vi "get_transport_error.vi"(8 "error in (no error)":errorcluster, 11 "Request in":refnum<class "Request.lvclass">) -> (0 "error out":errorcluster, 2 "transport_error":string, 3 "Request in":refnum<class "Request.lvclass">)   [LabVIEW 2020, in "reqwest.lvlib" / "Request.lvclass"]
uses:
  Request.lvclass
  Request.lvclass/Request.ctl
  reqwest.lvlib
  lv_reqwest_32.dll
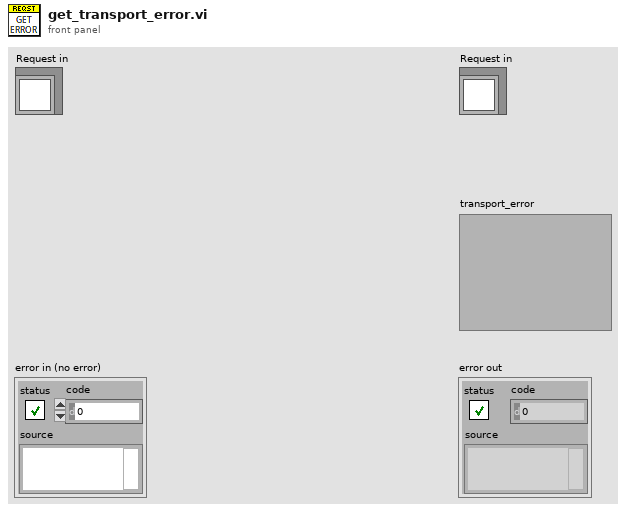
[diagram p1: front panel]
types:
  T1 = typedef "reqwest.lvlib/Request.lvclass/request_id.ctl" = u64
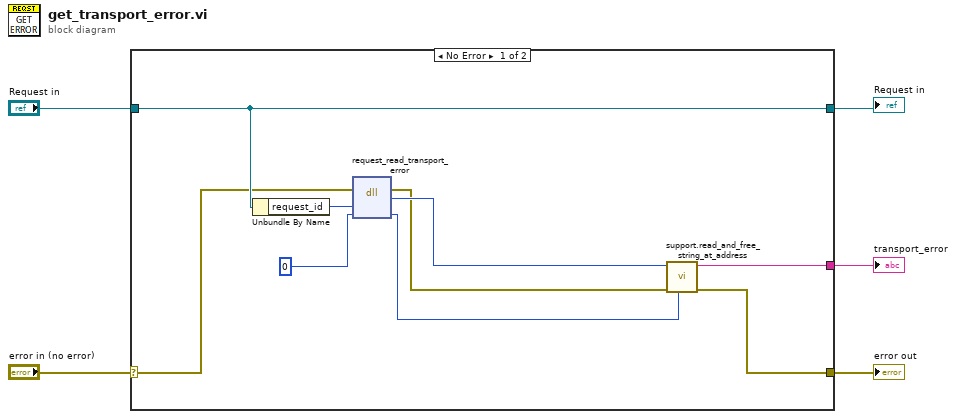
[diagram p0: block diagram]
diagram:
  n1 = case shown="No Error" "error in (no error)" {
    selector: "error in (no error)" -> [w9 w15]
    tunnel: "Request in" -> [w10 w16]
    tunnel: [w11 _] -> w3
    tunnel: [w8 w15] -> w1
    tunnel: [w10 w16] -> w2
    frame No Error {
      n2 = Unbundle By Name(w10) -> ("request_id"=w12:T1)
      n3 = dll-call lib="C:/Projects/reqwest-rs-labview/lv_src/lv_reqwest_*.*" fn="request_read_transport_error"(error in=w9, "request_id"=w12, "num_bytes"=u32 0) -> (error out=w13:errorcluster, "string_ptr"=w14:u64, "num_bytes"=w6:u32)  [unwired: 3 in, 1 out]
      n4 = call "support.read_and_free_string_at_address.vi"("string_length"=w6, "error in (no error)"=w13, "string_ptr"=w14) -> ("error out"=w8:errorcluster, "string"=w11:string)  [unwired: 7 in]
    }
    frame Error {
    }
  }
  "error out" <- w1
  "transport_error" <- w3
  "Request in" <- w2
